vi "read distance.vi"(8 "error in (no error)":errorcluster) -> (0 "error out":errorcluster, 5 "Distance 2":dbl)   [LabVIEW 2016]
uses:
  <vilib>/Rock Robotics/WPI/Ultrasonic/WPI_SonarMB1010AnalogRefNum Registry Get.vi
  <vilib>/Rock Robotics/WPI/Ultrasonic/WPI_SonarMB1010AnalogGetRange.vi
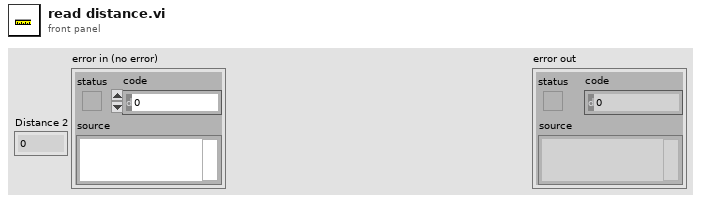
[diagram p1: front panel]
types:
  T1 = typedef "WPI_SonarMB1010AnalogDeviceRef.ctl" = cluster{"AIDeviceRef":T2, "Scaling factor (V/in)":dbl, "Average Bits":u8}
  T2 = typedef "WPI_AnalogChannelDevRef.ctl" = cluster{"DevStatus":errorcluster, "Analog Channel":T3}
  T3 = typedef "FPGA_AIChannel.ctl" = enum8{"AI 0", "AI 1", "AI 2", "AI 3", "AI MXP 0", "AI MXP 1", "AI MXP 2", "AI MXP 3", "Invalid"}
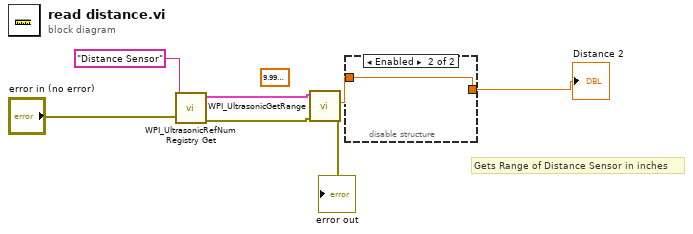
[diagram p0: block diagram]
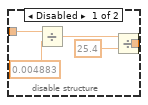
[diagram p2: hidden frame]
diagram:
  (unwired) sgl 1e-05 ("ping time (s)")
  # "Gets Range of Distance Sensor in inches"
  n1 = call-poly <vilib>:"WPI_UltrasonicRefNum Registry Get.vi"("error in (no error)"="error in (no error)", "refnum name"="Distance Sensor") -> ("error out"=w5:errorcluster, "SonarMB1010AnalogDevRef"=w6:T1)  [unwired: 8 in]
  n2 = call-poly <vilib>:"WPI_UltrasonicGetRange.vi"("error in"=w5, "SonarMB1010AnalogDevRef"=w6) -> ("error out"=→"error out":errorcluster, "Distance"=w2:dbl)  [unwired: 7 in, 1 out]
  n3 = disable-structure shown="Enabled" {
    disable-tunnel: w2 -> [w12 w13]
    disable-tunnel: [w8 w13] -> w1
    frame Disabled {
      n4 = Divide(x=w12, y=0.004883) -> (x/y=w10:dbl)
      n5 = Divide(x=w10, y=25.4) -> (x/y=w8:dbl)
    }
    frame Enabled {
    }
  }
  "Distance 2" <- w1
